vi "BNC555.evt call Chan Pulse.vi"(0 "i ref in":refnum<vi>, 2 "Generator Instance":string="N/A", 3 "Channel":i32(ring)=1 items=["System (To)", "Channel A", "Channel B", "Channel C", "Channel D", "Channel E", "Channel F", "Channel G", "Channel H"], 5 "error in (no error)":errorcluster, 7 "Delay":dbl format="%.6p", 9 "Width":dbl format="%.6p") -> (14 "i ref out":refnum<vi>, 19 "error out":errorcluster)   [LabVIEW 2014, in "BNC555.lvlib"]
doc: "This VI sends a simple event call to the wired BNC555."
uses:
  BNC555.lvlib
  CS_Core/CSSystem/CoreLib/CoreLib.double 2 byte array.vi
  CS_Core/CSSystem/CoreLib/CoreLib.int 2 byte array.vi
  CS_Core/CSSystem/CoreLib/CoreLib.lvlib
  CS_Core/BaseProcess/BaseProcess.lvlib
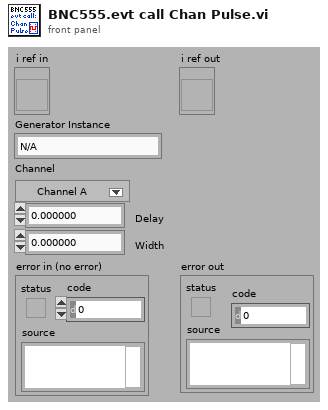
[diagram p1: front panel]
types:
  T1 = typedef "CoreDefs.rawDataType.ctl" = i8[]
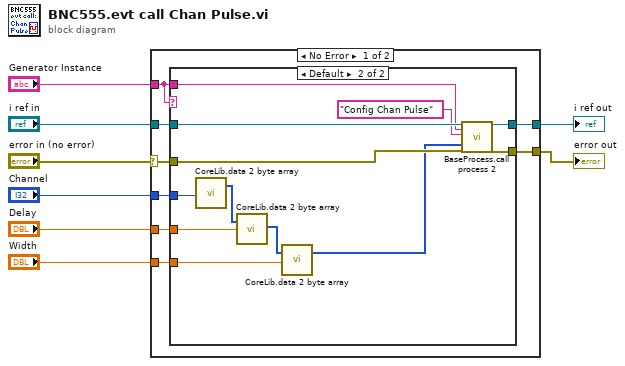
[diagram p0: block diagram]
diagram:
  n1 = case shown="No Error" "error in (no error)" {
    selector: "error in (no error)" -> [w13 w31]
    tunnel: [w16 w32] -> w7
    tunnel: [w15 w31] -> w6
    tunnel: "i ref in" -> [w14 w32]
    tunnel: "Generator Instance" -> [w12 _]
    tunnel: "Channel" -> [w11 _]
    tunnel: "Delay" -> [w10 _]
    tunnel: "Width" -> [w9 _]
    frame No Error {
      n2 = case shown="Default" w12 {
        tunnel: [w18 w30] -> w16
        tunnel: [w17 w29] -> w15
        tunnel: w14 -> [w18 w28]
        tunnel: w12 -> [_ w27]
        tunnel: w13 -> [w17 w25]
        tunnel: w11 -> [_ w24]
        tunnel: w10 -> [_ w23]
        tunnel: w9 -> [_ w20]
        frame "N/A" {
        }
        frame Default {
          n3 = call-poly "CoreLib.data 2 byte array.vi"("i32"=w24) -> ("byteArray out"=w22:T1)  [unwired: 18 in]
          n4 = call-poly "CoreLib.data 2 byte array.vi"("byteArray"=w22, "f64"=w23) -> ("byteArray out"=w21:T1)  [unwired: 17 in]
          n5 = call-poly "CoreLib.data 2 byte array.vi"("byteArray"=w21, "f64"=w20) -> ("byteArray out"=w19:T1)  [unwired: 17 in]
          n6 = call "BaseProcess.call process 2.vi"("i ref in"=w28, "Object"=w27, "Selector"="Config Chan Pulse", "Data"=w19, "error in (no error)"=w25) -> ("i ref out"=w30:refnum<vi>, "error out"=w29:errorcluster)  [unwired: 13 in]
        }
      }
    }
    frame Error {
    }
  }
  "error out" <- w6
  "i ref out" <- w7
